vi "Main FPGA.vi"() -> ()   [LabVIEW 2020]
uses:
  <vilib>/eio/EIONode/EIONode.xnode
  <vilib>/rvi/eio/common/nirviEmuTemplateMethod_errors.vi
panel:
  in  "Loop Time (ms)":u32=100 caption="Count(mSec)"
  in  "LED3":bool
  in  "LED2":bool
  in  "LED1":bool
  in  "LED0":bool
  out "AccelerationZ":i16
  out "AccelerationY":i16
  out "AccelerationX":i16
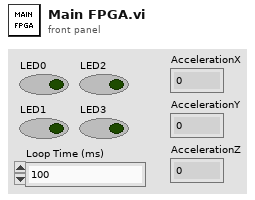
[diagram p1: front panel]
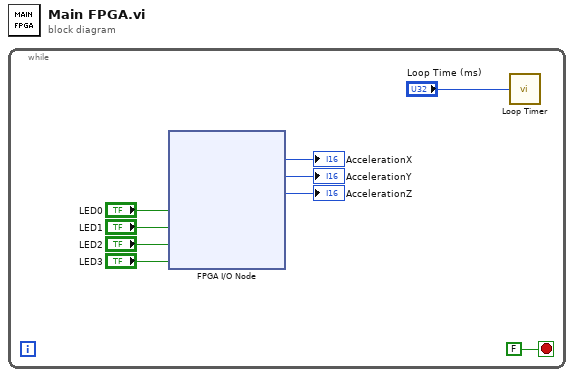
[diagram p0: block diagram]
diagram:
  n1 = while {
    stop <- FALSE stop-if-true
    n2 = xnode "FPGA I/O Node"("LED0"="LED0", "LED1"="LED1", "LED2"="LED2", "LED3"="LED3") -> ("AccelerationX"=→"AccelerationX":i16, "AccelerationY"=→"AccelerationY":i16, "AccelerationZ"=→"AccelerationZ":i16)  [unwired: 7 in, 7 out]
    n3 = call "Loop Timer"("Count(mSec)"="Loop Time (ms)") -> ()  [unwired: 1 out]
  }
